vi "5.2-4.7.2-Where Client.vi"() -> ()   [LabVIEW 2010]
doc: "This VI implements a client for the Named Service UDP Server.vi.\nIt connects to a service by specifying the server address and the name of the service. After sending a 'Hello' string to the server, the client receives the string sent by the server, displays the string and closes the connection.\n\n<b>Note:</b> This VI is built to work with the Named Service UDP Server.vi in UDP.llb.\nUDP Mutlicast Addressing Scheme:\n\n3.7 - Multicast Address: 224.0.3.7\n3.1-4.7.1 Port: 31471\n3.2-4.7.2 Port: 32472\n3.3-4.7.3 Port: 33473\n3.4-4.7.4 Port: 34474\n\n5.7 - Multicast Address: 224.0.5.7\n5.1-4.7.1 Port: 51471\n5.2-4.7.2 Port: 52472\n5.3-4.7.3 Port: 53473\n5.4-4.7.4 Port: 54474\n\n5.1-6.7.1 Port: 51671\n5.2-6.7.2 Port: 52672\n5.3-6.7.3 Port: 53673\n5.4-6.7.4 Port: 54674\n\n7.7 - Multicast Address: 224.0.7.7\n7.1-6.7.1 Port: 61671\n7.2-6.7.2 Port: 62672\n7.3-6.7.3 Port: 63673\n7.4-6.7.4 Port: 64674"
uses:
  4-High Neurons/4.2-Where Sensor Typedef.ctl
  4-High Neurons/Current GPS Data.ctl
  3-Midbrain/3.2-Where/_typedefs/3.2.1-VectorNav Data.ctl
  <vilib>/Utility/tcp.llb/UDP Multicast Open.vi
  5.0-Global.vi
  5.7-UDP/5.7-UDP Check Checksum.vi
  <vilib>/addons/internet/NI_InternetTK_Common_VIs.lvlib
panel:
  out "data":T1 {"4.2.2- Current GPS Data"."Longitude (dd.mmmmmm)" format="%#.6g"; "4.2.2- Current GPS Data"."Lattitude (dd.mmmmmm)" format="%#.6g"}
  out "Error":errorcluster
  in  "stop":bool
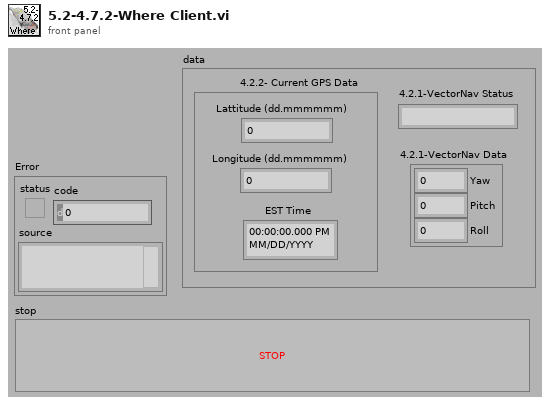
[diagram p1: front panel]
types:
  T1 = typedef "4.2-Where Sensor Typedef.ctl" = cluster{"4.2.2- Current GPS Data":T2, "4.2.1-VectorNav Data":T3, "4.2.1-VectorNav Status":string}
  T2 = typedef "Current GPS Data.ctl" = cluster{"Lattitude (dd.mmmmmm)":ext, "Longitude (dd.mmmmmm)":ext, "EST Time":timestamp}
  T3 = typedef "3.2.1-VectorNav Data.ctl" = cluster{"Yaw":dbl, "Pitch":dbl, "Roll":dbl}
  T4 = typedef "4.0-Timing Badass.ctl" = cluster{"Loop Period (ms)":u32, "HB":bool, "Last Time (ms)":u32, "Execution (ms)":u32}
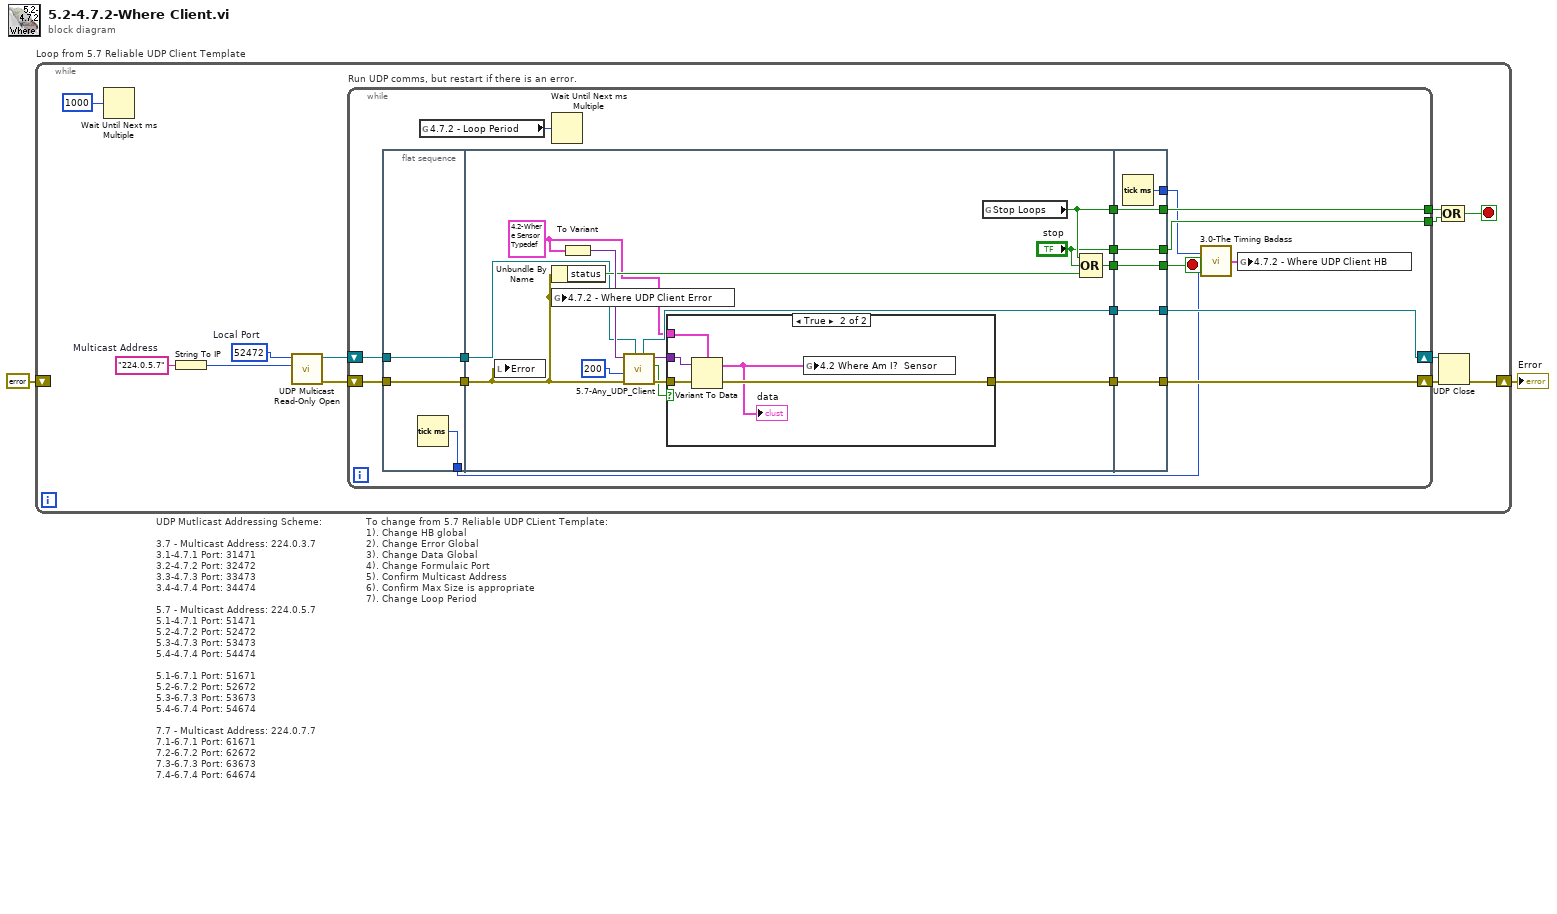
[diagram p0: block diagram]
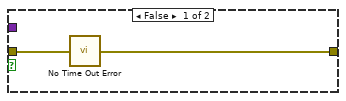
[diagram p2: hidden frame]
diagram:
  # "To change from 5.7 Reliable UDP CLient Template:\n1). Change HB global\n2). Change Error Global\n3). Change Data Global\n4). Change Formulaic Port\n5). Confirm Multicast Address\n6). Confirm Max Size is appropriate\n7). Change Loop Period"
  # "UDP Mutlicast Addressing Scheme:\n\n3.7 - Multicast Address: 224.0.3.7\n3.1-4.7.1 Port: 31471\n3.2-4.7.2 Port: 32472\n3.3-4.7.3 Port: 33473\n3.4-4.7.4 Port: 34474\n\n5.7 - Multicast Address: 224.0.5.7\n5.1-4.7.1 Port: 51471\n5.2-4.7.2 Port: 52472\n5.3-4.7.3 Port: 53473\n5.4-4.7.4 Port: 54474\n\n5.1-6.7.1 Port: 51671\n5.2-6.7.2 Port: 52672\n5.3-6.7.3 Port: 53673\n5.4-6.7.4 Port: 54674\n\n7.7 - Multicast Address: 224.0.7.7\n7.1-6.7.1 Port: 61671\n7.2-6.7.2 Port: 62672\n7.3-6.7.3 Port: 63673\n7.4-6.7.4 Port: 64674"
  n1 = while "Loop from 5.7 Reliable UDP Client Template" {
    shift-right: [w9] -> w2
    shift-left: errorcluster {"status"=FALSE, "code"=0, "source"=""} ("error out") -> [_]
    stop <- w12 stop-if-true
    w5 = u16 52472  # Local Port
    w7 = "224.0.5.7"  # Multicast Address
    n2 = Wait Until Next ms Multiple(millisecond multiple=u32 1000) -> ()  [unwired: 1 out]
    n3 = String To IP(1:w7) -> (0:w6:u32)
    n4 = call-poly <vilib>:"UDP Multicast Read-Only Open.vi"("multicast addr"=w6, "port"=w5) -> ("error out"=w3:errorcluster, "connection ID"=w4:refnum<k16>)  [unwired: 2 in, 6 out]
    n5 = while "Run UDP comms, but restart if there is an error." {
      tunnel: [w31] -> w14
      tunnel: [w30] -> w13
      shift-right: [w28] -> w11
      shift-left: w4 -> [w29]
      shift-right: [w27] -> w10
      shift-left: w3 -> [w26]
      stop <- w32 stop-if-true
      n6 = flat-sequence {
        tunnel: w26 -> [w34]
        tunnel: w29 -> [w35]
        tunnel: [w35] -> w19
        tunnel: [w34] -> w18
        tunnel: [w33] -> w16
        tunnel: [w49] -> w24
        tunnel: [w46] -> w23
        tunnel: ["stop"] -> w22
        tunnel: [w42] -> w21
        tunnel: [w41] -> w20
        tunnel: w19 -> [w43]
        tunnel: w18 -> [w38]
        tunnel: [w58] -> w27
        tunnel: [w59] -> w28
        tunnel: [w60] -> w30
        tunnel: [w61] -> w31
        tunnel: [w62] -> w32
        tunnel: w24 -> [w62]
        tunnel: w23 -> [w61]
        tunnel: w22 -> [w60]
        tunnel: w21 -> [w59]
        tunnel: w20 -> [w58]
        tunnel: [w57] -> w17
        frame #0 {
          n7 = Tick Count (ms)() -> (millisecond timer value=w33:u32)
        }
        frame #1 {
          w36 = T1 {"4.2.2- Current GPS Data"={"Lattitude (dd.mmmmmm)"=0.0, "Longitude (dd.mmmmmm)"=0.0, "EST Time"=timestamp(0 s since 1904-01-01)}, "4.2.1-VectorNav Data"={"Yaw"=0.0, "Pitch"=0.0, "Roll"=0.0}, "4.2.1-VectorNav Status"=""} ("data")
          n8 = local write "Error"(w38) -> ()
          n9 = Unbundle By Name(w38) -> ("status"=w44:bool)
          n10 = global write "5.0-Global.vi" "4.7.2 - Where UDP Client Error"(w38) -> ()
          n11 = To Variant(anything=w36) -> (Variant=w48:variant)
          n12 = call "5.7-Any_UDP_Client.vi"("Port In"=w43, "error In"=w38, "Max Size"=200, "DataTypeIn"=w48) -> ("Error Out"=w40:errorcluster, "Check Passed"=w39:bool, "DataOut"=w47:variant, "Port out"=w42:refnum<k16>)  [unwired: 4 in]
          n13 = case "Ignore Timeouts" shown="True" w39 {
            tunnel: w47 -> [_ w56]
            tunnel: w36 -> [_ w55]
            tunnel: w40 -> [w51 w54]
            tunnel: [w50 w53] -> w41
            frame False {
              n14 = call <vilib>:"No Time Out Error.vi"("error in (no error)"=w51) -> ("error out"=w50:errorcluster)  [unwired: 14 in]
            }
            frame True {
              n15 = Variant To Data(error in=w54, Variant=w56, type=w55) -> (error out=w53:errorcluster, data=w52:T1)
              "data" <- w52
              n16 = global write "5.0-Global.vi" "4.2 Where Am I?  Sensor"(w52) -> ()
            }
          }
          n17 = global read "5.0-Global.vi" "Stop Loops"() -> (w46:bool)
          n18 = Compound Arithmetic op=OR(w46, "stop", w44) -> (w49:bool)
        }
        frame #2 {
          n19 = Tick Count (ms)() -> (millisecond timer value=w57:u32)
        }
      }
      n20 = global read "5.0-Global.vi" "4.7.2 - Loop Period"() -> (w25:u32)
      n21 = Wait Until Next ms Multiple(millisecond multiple=w25) -> ()  [unwired: 1 out]
      n22 = call "3.0-The Timing Badass.vi"("Start"=w16, "End"=w17) -> ("Super Heart Beat"=w15:T4)
      n23 = global write "5.0-Global.vi" "4.7.2 - Where UDP Client HB"(w15) -> ()
    }
    n24 = UDP Close(connection ID=w11, 8:w10) -> (error out=w9:errorcluster)  [unwired: 1 out]
    n25 = Compound Arithmetic op=OR(w14, w13) -> (w12:bool)
  }
  "Error" <- w2
